vi "PiezoController.vi"() -> ()   [LabVIEW 2009]
uses:
  Controls/PIEZO.STATE.ctl
  Controls/PIEZO.COMMAND.ctl
  Controls/PIEZO.COMMANDBASIC.ctl
  Controls/PIEZO.WAVE.ctl
panel:
  out "Waveform":waveform(dbl)(graph)
  out "error out":errorcluster
  out "STATE":T1
  in  "PROCESS":string="PIEZO"
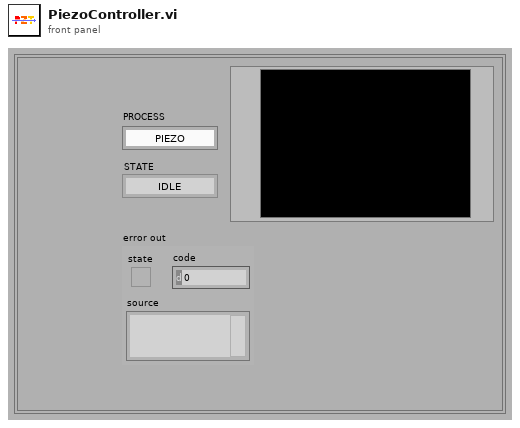
[diagram p1: front panel]
types:
  T1 = typedef "PIEZO.STATE.ctl" = enum16{"IDLE", "STARTING", "RUNNING", "STOPPING", "OFF"}
  T2 = typedef "PIEZO.COMMAND.ctl" = cluster{"Command":T3, "WAVE":T4}
  T3 = typedef "PIEZO.COMMANDBASIC.ctl" = enum16{"RUN", "STOP", "QUIT"}
  T4 = typedef "PIEZO.WAVE.ctl" = cluster{"Speed":dbl[unit], "Stiffness (0.95)":dbl, "Linear Stroke":dbl[unit], "Delay":dbl[unit]}
  T5 = typedef "PiezoSynchronization.ctl" = cluster{"COMMAND":T6, "STATE":refnum<notifier>, "WAVE":T7}
  T6 = typedef "PIEZO.COMMAND.QUEUE.ctl" = refnum<queue>
  T7 = typedef "PIEZO.WAVE.NOTIFIER.ctl" = refnum<notifier>
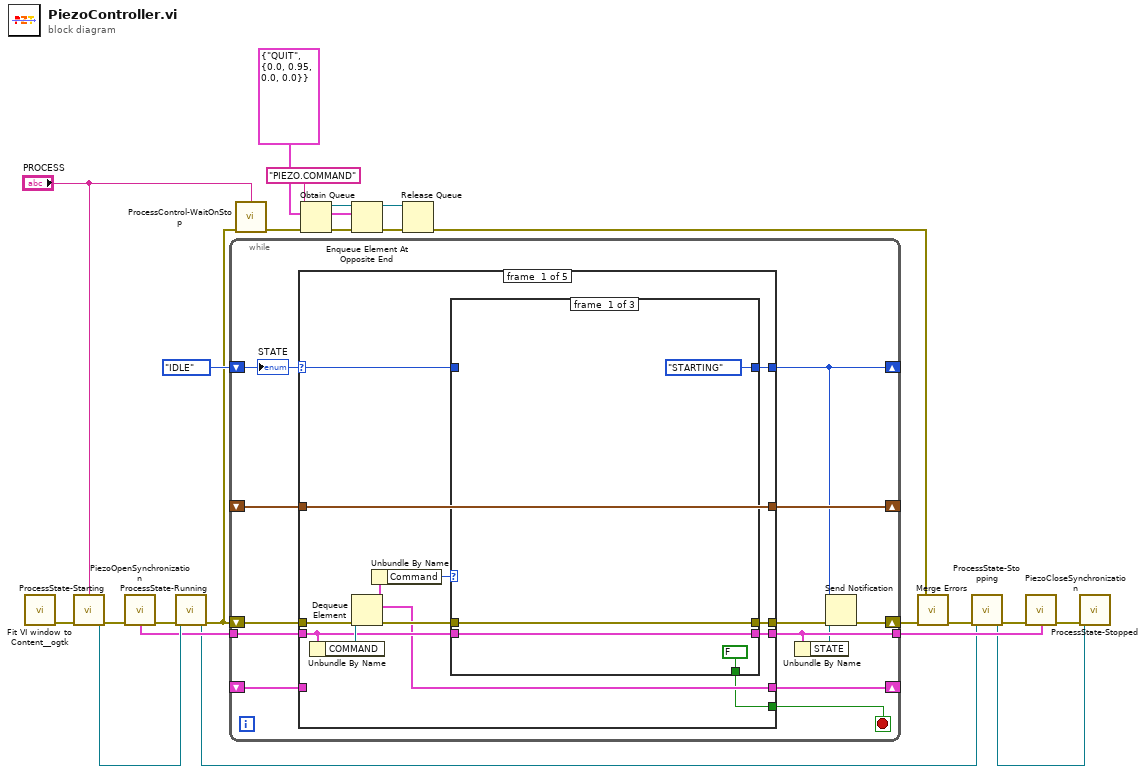
[diagram p0: block diagram]
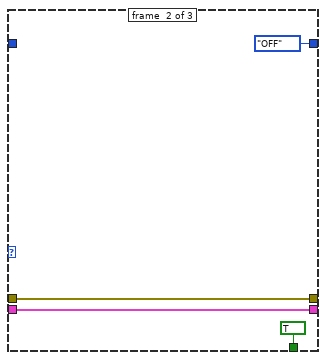
[diagram p2: hidden frame]
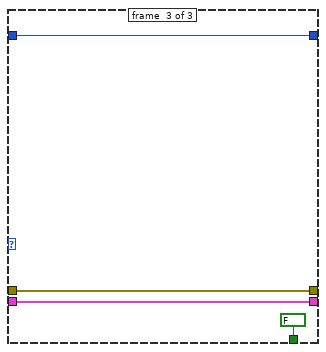
[diagram p3: hidden frame]
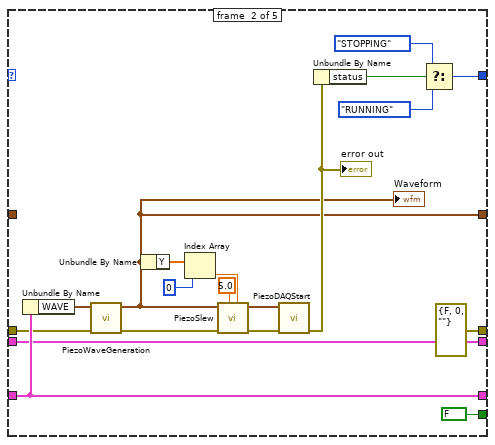
[diagram p4: hidden frame]
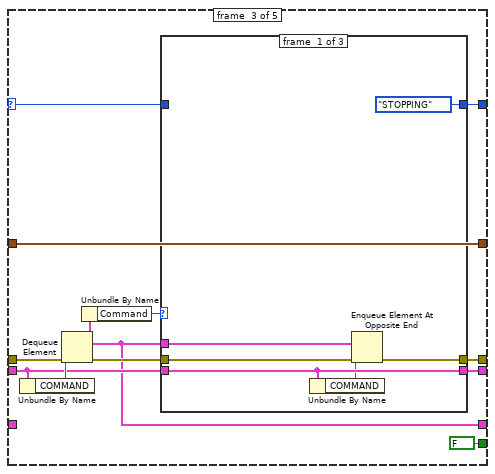
[diagram p5: hidden frame]
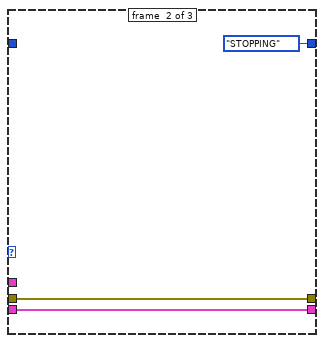
[diagram p6: hidden frame]
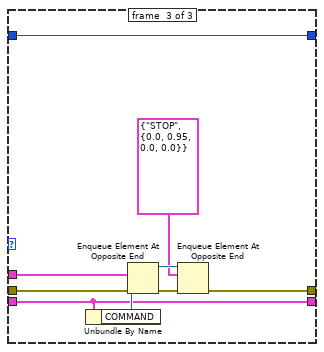
[diagram p7: hidden frame]
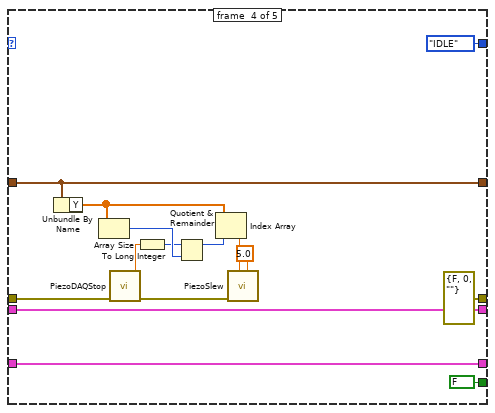
[diagram p8: hidden frame]
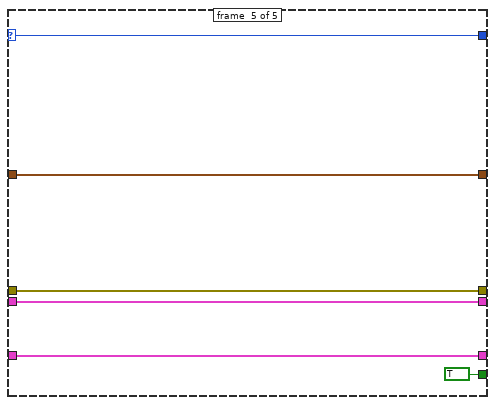
[diagram p9: hidden frame]
diagram:
  w8 = T2 {"Command"=enum."QUIT", "WAVE"={"Speed"=0.0, "Stiffness (0.95)"=0.95, "Linear Stroke"=0.0, "Delay"=0.0}} ("COMMAND")
  n1 = call <userlib>:"Fit VI window to Content__ogtk.vi"() -> ("error out"=w1:errorcluster)  [unwired: 6 in, 1 out]
  n2 = call "ProcessState-Starting.vi"("PROCESS"="PROCESS", "error in (no error)"=w1) -> ("ProcessStateNotifier"=w20:refnum<notifier>, "error in (no error)"=w22:errorcluster)  [unwired: 6 in]
  n3 = call "PiezoOpenSynchronization.vi"("error in (no error)"=w22) -> ("error out"=w21:errorcluster, "PiezoSynchronization"=w19:T5)  [unwired: 7 in]
  n4 = call "ProcessState-Running.vi"("ProcessStateNotifier in"=w20, "error in (no error)"=w21) -> ("ProcessStateNotifier out"=w15:refnum<notifier>, "error out"=w13:errorcluster)  [unwired: 6 in]
  n5 = while {
    shift-right: [w24] -> _
    shift-left: PIEZO.STATE."IDLE" ("STATE") -> [w34]
    shift-right: [w28] -> w5
    shift-left: w13 -> [w36]
    tunnel: w19 -> [w35]
    shift-right: [w33] -> _
    shift-left: _ -> [w32]
    tunnel: [w26] -> w16
    shift-right: [w31] -> _
    shift-left: _ -> [w30]
    stop <- w29 stop-if-true
    n6 = case shown="\"STOPPING\"" w34 {
      selector: w34 -> [w43 _ w85 _ w129]
      tunnel: w36 -> [w48 w76 w90 w120 w127]
      tunnel: w35 -> [w45 w75 w87 w121 w126]
      tunnel: [w41 w78 w81 w122 w125] -> w33
      tunnel: w32 -> [_ w78 _ w122 w125]
      tunnel: [w42 w70 w84 PIEZO.STATE."IDLE" ("STATE") w129] -> w24
      tunnel: [w40 errorcluster {"status"=FALSE, "code"=0, "source"=""} ("error out") w83 errorcluster {"status"=FALSE, "code"=0, "source"=""} ("error out") w127] -> w27
      tunnel: [w39 w75 w82 w121 w126] -> w26
      tunnel: [w38 FALSE FALSE FALSE TRUE] -> w29
      tunnel: [w37 w61 w79 w115 w128] -> w31
      tunnel: w30 -> [w37 _ w79 w115 w128]
      frame #0 {
        n7 = Unbundle By Name(w45) -> ("COMMAND"=w47:T6)
        n8 = Dequeue Element(queue=w47, error in (no error)=w48) -> (element=w41:T2, error out=w44:errorcluster)  [unwired: 1 in, 2 out]
        n9 = Unbundle By Name(w41) -> ("Command"=w46:T3)
        n10 = case shown="\"QUIT\"" w46 {
          tunnel: w45 -> [w50 w55 w59]
          tunnel: w44 -> [w51 w56 w60]
          tunnel: w43 -> [_ _ w57]
          tunnel: [PIEZO.STATE."STARTING" ("STATE") PIEZO.STATE."OFF" ("STATE") w57] -> w42
          tunnel: [w51 w56 w60] -> w40
          tunnel: [w50 w55 w59] -> w39
          tunnel: [FALSE TRUE FALSE] -> w38
          frame #0 {
          }
          frame #1 {
          }
          frame #2 {
          }
        }
      }
      frame #1 {
        n11 = Unbundle By Name(w78) -> ("WAVE"=w77:T4)
        n12 = call "PiezoWaveGeneration.vi"("WAVE"=w77, "error in (no error)"=w76) -> ("Graphe"=w61:waveform(dbl), "error out"=w66:errorcluster)  [unwired: 6 in]
        "Waveform" <- w61
        n13 = Unbundle By Name(w61) -> ("Y"=w64:dbl[])
        n14 = Index Array(array=w64, index=0 ("indice")) -> (element=w63:dbl)
        n15 = call "PiezoSlew.vi"("To"=w63, "From"=5.0, "error in (no error)"=w66) -> ("error out"=w65:errorcluster)  [unwired: 6 in]
        n16 = call "PiezoDAQStart.vi"("Waveform"=w61, "error in (no error)"=w65) -> ("error out"=w73:errorcluster)  [unwired: 8 in]
        "error out" <- w73
        n17 = Unbundle By Name(w73) -> ("status"=w72:bool)
        n18 = Select(t=PIEZO.STATE."STOPPING" ("STATE"), s=w72, f=PIEZO.STATE."RUNNING" ("STATE")) -> (s? t:f=w70:T1)
      }
      frame #2 {
        n19 = Unbundle By Name(w87) -> ("COMMAND"=w89:T6)
        n20 = Dequeue Element(queue=w89, error in (no error)=w90) -> (element=w81:T2, error out=w86:errorcluster)  [unwired: 1 in, 2 out]
        n21 = Unbundle By Name(w81) -> ("Command"=w88:T3)
        n22 = case shown="\"STOP\"" w88 {
          tunnel: w87 -> [w93 w97 w106]
          tunnel: w86 -> [w95 w98 w105]
          tunnel: w85 -> [_ _ w108]
          tunnel: [PIEZO.STATE."STOPPING" ("STATE") PIEZO.STATE."STOPPING" ("STATE") w108] -> w84
          tunnel: [w94 w98 w100] -> w83
          tunnel: [w93 w97 w106] -> w82
          tunnel: w81 -> [w91 _ w102]
          frame #0 {
            n23 = Unbundle By Name(w93) -> ("COMMAND"=w92:T6)
            n24 = Enqueue Element At Opposite End(queue=w92, element=w91, error in (no error)=w95) -> (error out=w94:errorcluster)  [unwired: 1 in, 2 out]
          }
          frame #1 {
          }
          frame #2 {
            n25 = Unbundle By Name(w106) -> ("COMMAND"=w107:T6)
            n26 = Enqueue Element At Opposite End(queue=w107, element=w102, error in (no error)=w105) -> (queue out=w103:T6, error out=w104:errorcluster)  [unwired: 1 in, 1 out]
            n27 = Enqueue Element At Opposite End(queue=w103, element=T2 {"Command"=enum."STOP", "WAVE"={"Speed"=0.0, "Stiffness (0.95)"=0.95, "Linear Stroke"=0.0, "Delay"=0.0}} ("élément"), error in (no error)=w104) -> (error out=w100:errorcluster)  [unwired: 1 in, 2 out]
          }
        }
      }
      frame #3 {
        n28 = Unbundle By Name(w115) -> ("Y"=w111:dbl[])
        n29 = Array Size(array=w111) -> (size(s)=w113:i32)
        n30 = call "PiezoDAQStop.vi"("error in (no error)"=w120) -> ("Last Value"=w114:dbl, "error out"=w117:errorcluster)  [unwired: 7 in]
        n31 = To Long Integer(number=w114) -> (32bit integer=w112:i32)
        n32 = Quotient & Remainder(x=w112, y=w113) -> (x-y*floor(x/y)=w110:i32)  [unwired: 1 out]
        n33 = Index Array(array=w111, index=w110) -> (element=w109:dbl)
        n34 = call "PiezoSlew.vi"("To"=5.0, "From"=w109, "error in (no error)"=w117) -> ()  [unwired: 6 in, 1 out]
      }
      frame #4 {
      }
    }
    n35 = Unbundle By Name(w26) -> ("STATE"=w25:refnum<notifier>)
    n36 = Send Notification(notification=w24, notifier=w25, error in (no error)=w27) -> (error out=w28:errorcluster)  [unwired: 1 out]
    "STATE" <- w34
  }
  n37 = call "ProcessControl-WaitOnStop.vi"("PROCESS"="PROCESS", "error out"=w13) -> ("error in"=w12:errorcluster)  [unwired: 7 in]
  n38 = Obtain Queue(name (unnamed)="PIEZO.COMMAND" ("nom (aucun)"), element data type=w8, error in (no error)=w12) -> (queue out=w9:refnum<queue>, error out=w10:errorcluster)  [unwired: 2 in, 1 out]
  n39 = Enqueue Element At Opposite End(queue=w9, element=w8, error in (no error)=w10) -> (queue out=w6:refnum<queue>, error out=w7:errorcluster)  [unwired: 1 in, 1 out]
  n40 = Release Queue(queue=w6, error in (no error)=w7) -> (error out=w3:errorcluster)  [unwired: 1 in, 2 out]
  n41 = call <vilib>:"Merge Errors.vi"("error in 3 (no error)"=w5, "error in 1 (no error)"=w3) -> ("error out"=w4:errorcluster)  [unwired: 5 in]
  n42 = call "ProcessState-Stopping.vi"("ProcessStateNotifier in"=w15, "error in (no error)"=w4) -> ("ProcessStateNotifier out"=w14:refnum<notifier>, "error out"=w18:errorcluster)  [unwired: 6 in]
  n43 = call "PiezoCloseSynchronization.vi"("PiezoSynchronization"=w16, "error in (no error)"=w18) -> ("error out"=w17:errorcluster)  [unwired: 7 in]
  n44 = call "ProcessState-Stopped.vi"("ProcessStateNotifier in"=w14, "error in (no error)"=w17) -> ()  [unwired: 7 in, 1 out]
